vi "AddAttribute.vi"(6 "Overwrite? (F)":bool, 8 "error in (no error)":errorcluster, 10 "Attribute":refnum<class "Attribute.lvclass">, 11 "SMO in":refnum<class "SMO.lvclass">) -> (0 "error out":errorcluster, 3 "SMO out":refnum<class "SMO.lvclass">)   [LabVIEW 2013, in "SMO.lvclass"]
uses:
  SMO.lvclass
  Support/Attribute/Attribute.lvclass
  SMO.lvclass/SMO.ctl
  Support/Attribute/Attribute.lvclass/Attribute.ctl
  <vilib>/Utility/LVClass/Get LV Class Name.vi
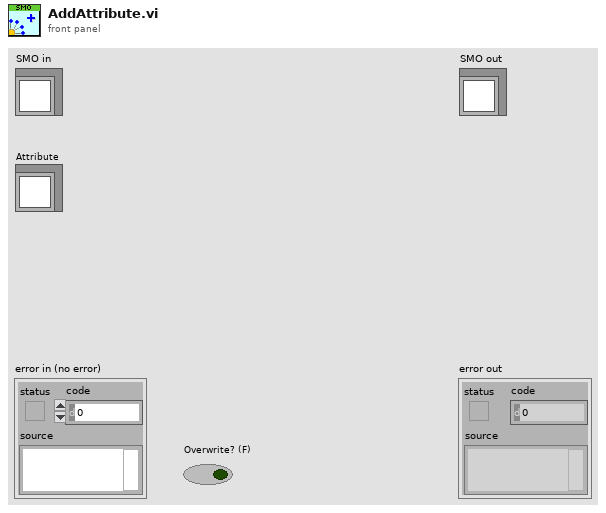
[diagram p1: front panel]
types:
  T1 = typedef "SMO.lvclass/PrivateData--Ref.ctl" = refnum<data-value>
  T2 = typedef "SMO.lvclass/PrivateData--Cluster.ctl" = cluster{"Parent Call":T3, "Registered Processes":T4[], "Sync Notifier":refnum<notifier>, "Process Error Notifier":refnum<notifier>, "Protected Events":T5, "Public Events":T6, "SMO State":T7, "[Dependencies]":T8[], "[Attributes]":variant, "Launcher Close":refnum<notifier>, "Caller Watchdog":refnum<queue>, "Accessibility":T9, "NbStaticDependencies":u32}
  T3 = typedef "SMO.lvclass/Parent Call--Enum.ctl" = enum16{"Allows parent to run", "Does not request parent to run"}
  T4 = typedef "SMO.lvclass/RegisteredProcessData--Cluster.ctl" = cluster{"Name":string, "Static VI Ref":refnum<vi>, "Running":bool, "NotifierRef":u32}
  T5 = typedef "SMO.lvclass/Protected Events.ctl" = cluster{"StopProcesses":refnum<user-event>, "AbortProcesses":refnum<user-event>, "Config Changed":refnum<user-event>, "Dependency":refnum<user-event>}
  T6 = typedef "SMO.lvclass/Public Events.ctl" = cluster{"Error":refnum<user-event>, "State":refnum<user-event>, "Reserve State":refnum<user-event>}
  T7 = typedef "SMO.lvclass/SMOState --Enum.ctl" = enum16{"unknown", "Created", "Started", "Stopped"}
  T8 = typedef "SMO.lvclass/SMO Dependency--Cluster.ctl" = cluster{"Dependency":refnum<class "SMO.lvclass">, "Level":string}
  T9 = typedef "SMO.lvclass/Accessibility--Cluster.ctl" = cluster{"Lock Key":string, "Reserve State":T10}
  T10 = typedef "SMO.lvclass/Reserve State--Enum.ctl" = enum16{"Unreserved", "Reserved", "Self-locked"}
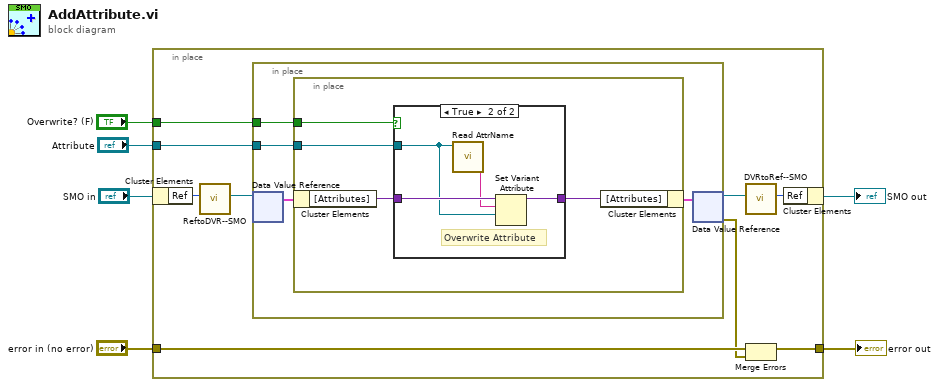
[diagram p0: block diagram]
diagram:
  n1 = in-place {
    in-place-border: "error in (no error)" -> [w11]
    in-place-border: [w9] -> w5
    in-place-border: "Attribute" -> [w8]
    in-place-border: "Overwrite? (F)" -> [w7]
    n2 = in-place-cluster #1("SMO in") -> ("Ref"=w15:u32)
    n3 = call "ReftoDVR--SMO.vi"("Ref"=w15) -> ("Ref"=w14:T1)  [unwired: 10 in]
    n4 = in-place {
      in-place-border: w8 -> [w19]
      in-place-border: w7 -> [w16]
      n5 = in-place-dvr #2(w14) -> (w18:T2)  [unwired: 1 out]
      n6 = in-place {
        in-place-border: w19 -> [w21]
        in-place-border: w16 -> [w20]
        n7 = in-place-cluster #3(w18) -> ("[Attributes]"=w23:variant)
        n8 = case shown="True" w20 {
          tunnel: w23 -> [w24 w28]
          tunnel: [w24 w27] -> w22
          tunnel: w21 -> [_ w26]
          frame False {
            # "Do not overwrite\nattribute"
          }
          frame True {
            # "Overwrite Attribute"
            n9 = call "Read AttrName.vi"("Attribute in"=w26) -> ("Attribute Name"=w25:string)  [unwired: 9 in, 1 out]
            n10 = Set Variant Attribute(Variant=w28, name=w25, value=w26) -> (Variant out=w27:variant)  [unwired: 1 in, 2 out]
          }
        }
        n11 = in-place-cluster #3("[Attributes]"=w22) -> (w17:T2)
      }
      n12 = in-place-dvr #2(w17) -> (w13:T1, w10:errorcluster)
    }
    n13 = call "DVRtoRef--SMO.vi"("Ref"=w13) -> ("Ref"=w12:u32)  [unwired: 10 in]
    n14 = Merge Errors(w11, w10) -> (w9:errorcluster)
    n15 = in-place-cluster #1("Ref"=w12) -> (→"SMO out":refnum<class "SMO.lvclass">)
  }
  "error out" <- w5
